vi "Write Float Configuration.vi"(7 "Type":T1, 8 "error in (no error)":errorcluster, 9 "Value":ext, 10 "Name":string, 11 "IniFileSection in":refnum<class "IniFileSection.lvclass">) -> (0 "error out":errorcluster, 3 "IniFileSection out":refnum<class "IniFileSection.lvclass">)   [LabVIEW 2020, in "IniFileSection.lvclass"]
uses:
  <vilib>/gpm_packages/@cs/Configuration/Source/IniFileSection/IniFileSection.lvclass
  <vilib>/Utility/Data Type/Type Definitions/Data Type.ctl
  <vilib>/gpm_packages/@cs/Configuration/Source/IniFileSection/IniFileSection.lvclass/IniFileSection.ctl
  <vilib>/Utility/config.llb/NI_LVConfig.lvlib
  <vilib>/Utility/Data Type/NI_Data Type.lvlib
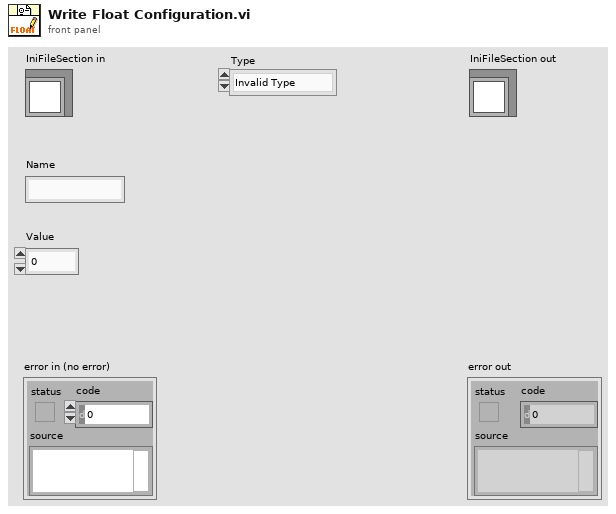
[diagram p1: front panel]
types:
  T1 = typedef "NI_Data Type.lvlib/Data Type.ctl" = enum8{"Invalid Type", "Void", "I8", "I16", "I32", "I64", "U8", "U16", "U32", "U64", "Single Float", "Double Float", "Extended Float", "Single Complex", "Double Complex", "Extended Complex", "Enum U8", "Enum U16", "Enum U32", "Enum U64", "Single Float With Unit", "Double Float With Unit", "Extended Float With Unit", "Single Complex with Unit", "Double Complex with Unit", "Extended Complex with Unit", "Boolean", "String", "Path", "Picture", "Tag", "Array", "Cluster", "Variant", "LV Variant", "Waveform", "Timestamp", "Digital Waveform", "Digital Data", "ExpressData", "Refnum", "External Data", "VI", "Poly VI", "LabVIEW Class Instance", "Fixed Point", "Set Collection", "Map Collection"}
  T2 = typedef "NI_LVConfig.lvlib/Config Data RefNum.ctl" = refnum<k1>
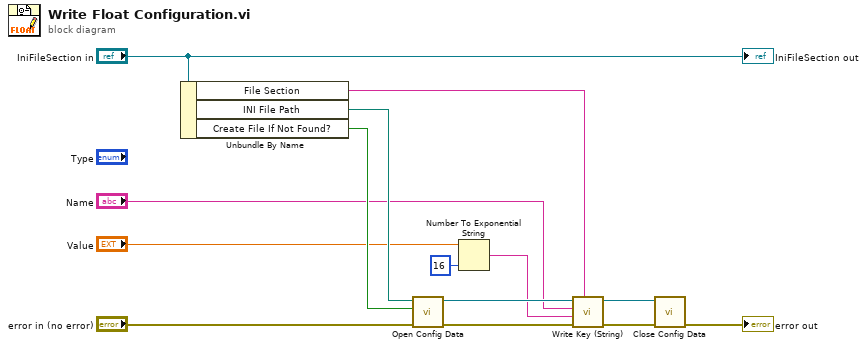
[diagram p0: block diagram]
diagram:
  n1 = Unbundle By Name("IniFileSection in") -> ("File Section"=w2:string, "INI File Path"=w13:path, "Create File If Not Found?"=w12:bool)
  n2 = call <vilib>:"Open Config Data.vi"("error in (no error)"="error in (no error)", "create file if necessary (T)"=w12, "configuration file path"=w13) -> ("error out"=w7:errorcluster, "refnum"=w14:T2)  [unwired: 6 in, 1 out]
  n3 = Number To Exponential String(number="Value", precision (6)=i16 16) -> (E-format string=w8:string)  [unwired: 2 in]
  n4 = call <vilib>:"Write Key (String).vi"("section"=w2, "error in (no error)"=w7, "value"=w8, "key"="Name", "refnum"=w14) -> ("error out"=w5:errorcluster, "refnum out"=w6:T2)  [unwired: 4 in, 1 out]
  n5 = call <vilib>:"Close Config Data.vi"("error in (no error)"=w5, "refnum"=w6) -> ("error out"=→"error out":errorcluster)  [unwired: 8 in, 1 out]
  "IniFileSection out" <- "IniFileSection in"
